vi "Remove Item.vi"(8 "error in (no error)":errorcluster, 11 "Listbox Refs in":T1 {"Section Ref" format="%.0x"}) -> (0 "error out":errorcluster, 3 "Listbox Refs out":T1 {"Section Ref" format="%.0x"})   [LabVIEW 2013, in "FPGA Addon System Explorer.lvlib"]
uses:
  FPGA Addon System Explorer.lvlib
  Listbox Cluster.ctl
  <vilib>/NI Veristand/Custom Device API/Custom Device Item Ref.ctl
  Shared/Constants.vi
  <vilib>/NI VeriStand/Custom Device API/Custom Device API.lvlib
  Shared/FPGA Addon Shared.lvlib
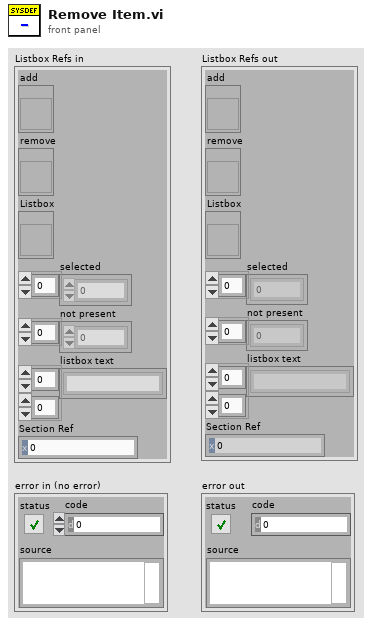
[diagram p1: front panel]
types:
  T1 = typedef "FPGA Addon System Explorer.lvlib/Listbox Cluster.ctl" = cluster{"add":refnum<vi>, "remove":refnum<vi>, "Listbox":refnum<vi>, "selected":i32[], "not present":i32[], "listbox text":string[][], "Section Ref":T2}
  T2 = typedef "Custom Device API.lvlib/Custom Device Item Ref.ctl" = u64
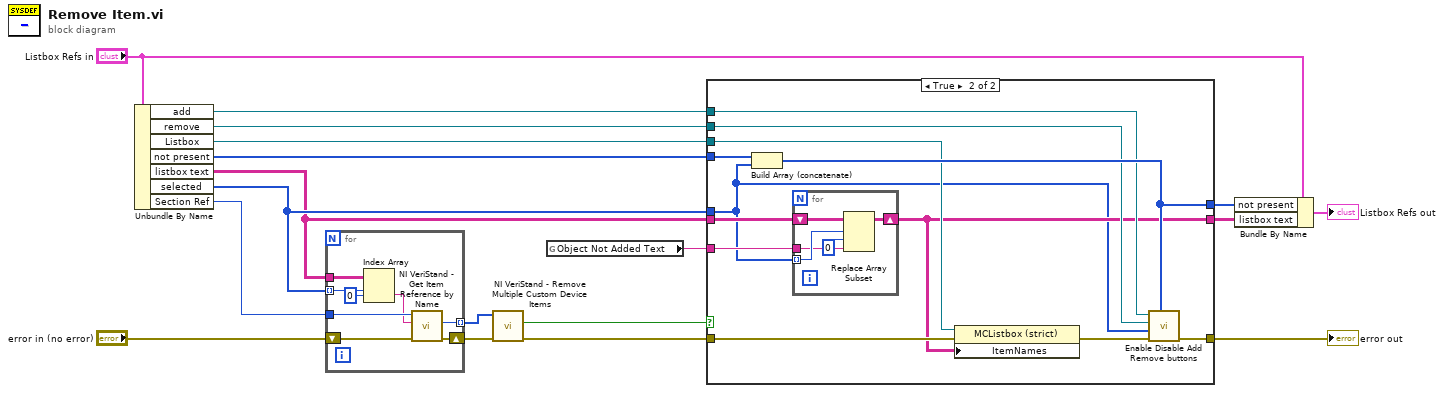
[diagram p0: block diagram]
diagram:
  n1 = Unbundle By Name("Listbox Refs in") -> ("add"=w3:refnum<vi>, "remove"=w2:refnum<vi>, "Listbox"=w1:refnum<vi>, "not present"=w13:i32[], "listbox text"=w4:string[][], "selected"=w5:i32[], "Section Ref"=w18:T2)
  n2 = for {
    tunnel: w5 -> [w25] mode=indexing
    tunnel: w4 -> [w26]
    tunnel: w18 -> [w22]
    tunnel: [w19] -> w9 mode=indexing
    shift-right: [w21] -> w10
    shift-left: "error in (no error)" -> [w23]
    n3 = Index Array(array=w26, index (row)=w25, index (col)=0 ("disabled index (col)")) -> (element=w20:string)
    n4 = call <vilib>:"NI VeriStand - Get Item Reference by Name.vi"("error in (no error)"=w23, "Item Name"=w20, "Parent Ref in"=w22) -> ("error out"=w21:errorcluster, "Item Ref"=w19:T2)  [unwired: 5 in, 2 out]
  }
  n5 = call <vilib>:"NI VeriStand - Remove Multiple Custom Device Items.vi"("error in (no error)"=w10, "Item Refs in"=w9) -> ("error out"=w8:errorcluster, "Deleted?"=w7:bool)  [unwired: 8 in]
  n6 = global read "Constants.vi" "Object Not Added Text"() -> (w6:string)
  n7 = case shown="True" w7 {
    tunnel: [w28 w41] -> w11
    tunnel: w8 -> [w28 w36]
    tunnel: w5 -> [_ w30]
    tunnel: w4 -> [w29 w40]
    tunnel: w6 -> [_ w39]
    tunnel: [w29 w31] -> w16
    tunnel: w13 -> [w27 w38]
    tunnel: [w27 w37] -> w15
    tunnel: w3 -> [_ w34]
    tunnel: w2 -> [_ w33]
    tunnel: w1 -> [_ w32]
    frame False {
    }
    frame True {
      n8 = Build Array (concatenate)(w38, w30) -> (w37:i32[])
      n9 = for {
        tunnel: w30 -> [w44] mode=indexing
        shift-right: [w45] -> w31
        shift-left: w40 -> [w46]
        tunnel: w39 -> [w42]
        n10 = Replace Array Subset(array=w46, new element=w42, index (row)=w44, index (col)=0 ("disabled index (col)")) -> (w45:string[][])
      }
      n11 = property class="MCListbox (strict)"(reference=w32, error in=w36, "ItemNames"=w31) -> (error out=w35:errorcluster)  [unwired: 1 out]
      n12 = call "Enable Disable Add Remove buttons.vi"("not present item indexes"=w37, "error in (no error)"=w35, "selected items"=w30, "remove button"=w33, "add button"=w34) -> ("error out"=w41:errorcluster)  [unwired: 6 in]
    }
  }
  "error out" <- w11
  n13 = Bundle By Name(cluster="Listbox Refs in", "not present"=w15, "listbox text"=w16) -> (→"Listbox Refs out":T1)
